vi "PMTlargeView.vi"(10 "queue in":refnum<queue>, 11 "PMT chart":cluster{"Frequency Chart":u32, "mean":dbl}(graph)) -> ()   [LabVIEW 2017]
uses:
  controls/ImagingStatusControl.ctl
  GlobalImagingStatus.vi
  Global.lvlib
panel:
  in  "stop":bool
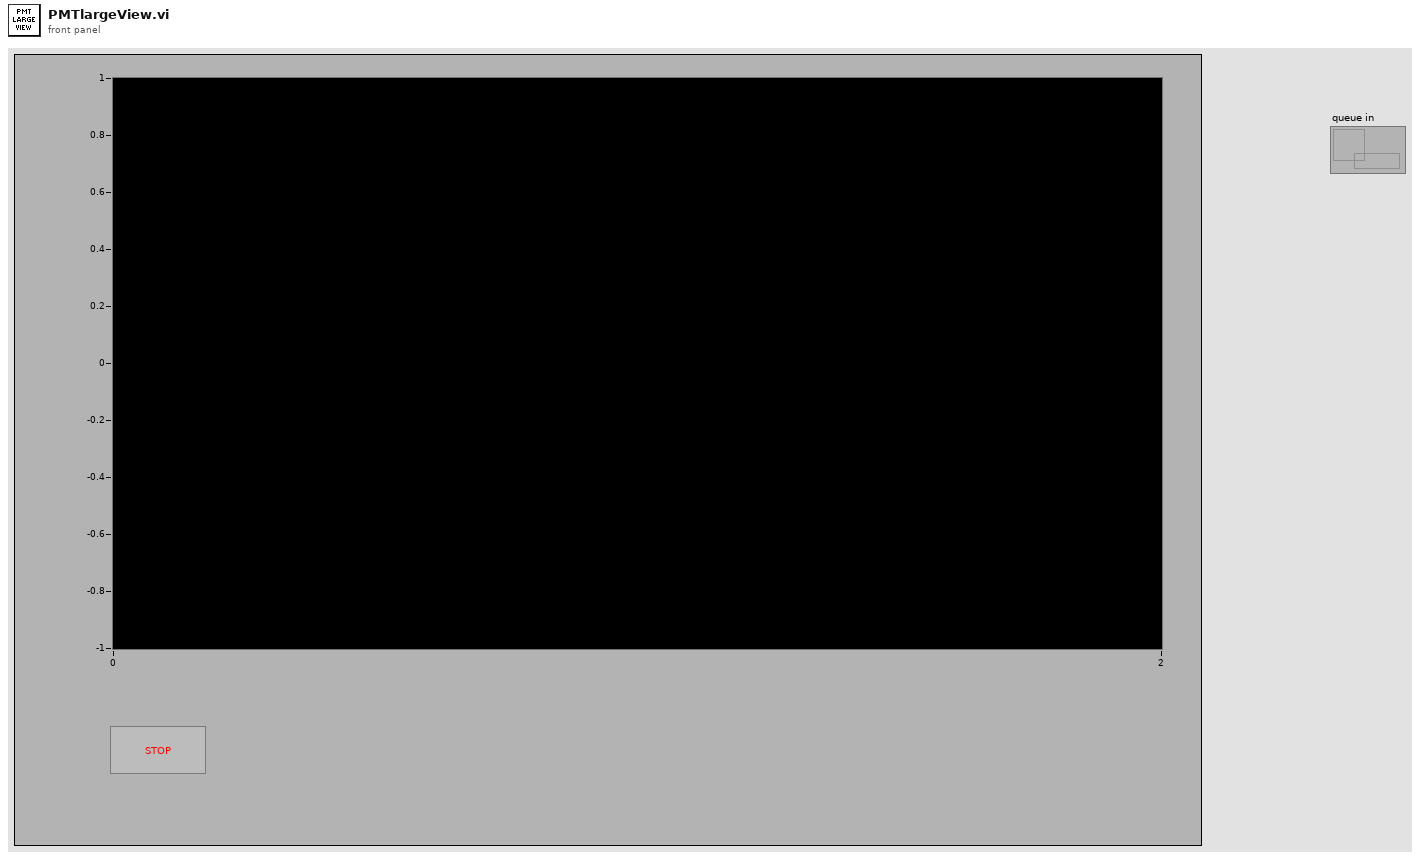
[diagram p1: front panel]
types:
  T1 = typedef "ImagingStatusControl.ctl" = enum16{"PMT_large", "Camera_large", "PMT", "Camera", "Idle"}
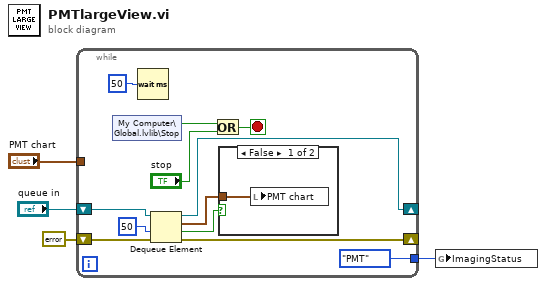
[diagram p0: block diagram]
diagram:
  n1 = while {
    tunnel: "PMT chart" -> [_]
    shift-right: [w11] -> _
    shift-left: "queue in" -> [w12]
    shift-right: [w9] -> _
    shift-left: errorcluster {"status"=FALSE, "code"=0, "source"=""} ("error out") -> [w10]
    tunnel: [ImagingStatusControl."PMT" ("ImagingStatus")] -> w1
    stop <- w14 stop-if-true
    n2 = shared-variable "My Computer\\Global.lvlib\\Stop"() -> (w16:bool)  [unwired: 1 in, 1 out]
    n3 = Wait (ms)(milliseconds to wait=u32 50) -> ()  [unwired: 1 out]
    n4 = Dequeue Element(queue=w12, timeout in ms (-1)=50, error in (no error)=w10) -> (queue out=w11:refnum<queue>, element=w13:cluster{dbl, dbl}, timed out?=w5:bool, error out=w9:errorcluster)
    n5 = Or(x=w16, y="stop") -> (x .or. y?=w14:bool)
    n6 = case shown="False" w5 {
      tunnel: w13 -> [w17 _]
      frame False {
        n7 = local write "PMT chart"(w17) -> ()
      }
      frame True {
      }
    }
  }
  n8 = global write "GlobalImagingStatus.vi" "ImagingStatus"(w1) -> ()
